vi "Get Communication Specific Objects.vi"(8 "error in":errorcluster, 11 "Electronic Datasheet":refnum<class "Electronic Datasheet.lvclass">) -> (0 "error out":errorcluster, 2 "Entries":refnum<class "OD Entry.lvclass">[](array[class]), 3 "Electronic Datasheet":refnum<class "Electronic Datasheet.lvclass">)   [LabVIEW 2024, in "Electronic Datasheet.lvlib" / "Electronic Datasheet.lvclass"]
uses:
  Electronic Datasheet.lvclass
  Core/OD Entry/OD Entry.lvclass
  Core/Sorted Object Dictionary/Sorted Object Dictionary.lvclass
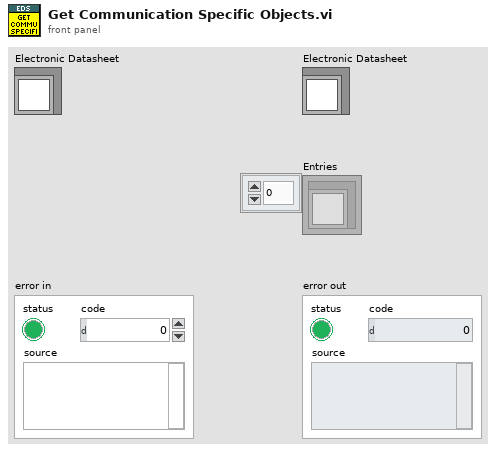
[diagram p1: front panel]
types:
  T1 = typedef "Electronic Datasheet.lvlib/Electronic Datasheet.lvclass/ObjectAttributes.ctl" = cluster{"EDS File Path":path, "Object Dict":refnum<class "Dictionary.lvclass">, "Sorted Object Dict":refnum<class "Sorted Object Dictionary.lvclass">, "Device Info":refnum<class "Device Info.lvclass">, "File Info":refnum<class "File Info.lvclass">}
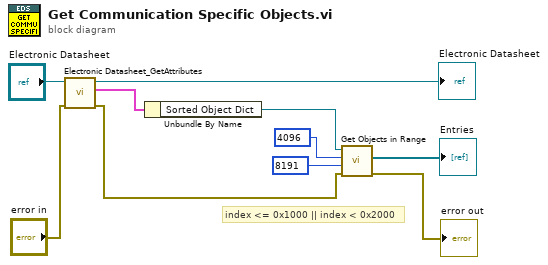
[diagram p0: block diagram]
diagram:
  # "index <= 0x1000 || index < 0x2000"
  n1 = call "Electronic Datasheet_GetAttributes.vi"("Error In"="error in", "reference in"="Electronic Datasheet") -> ("Error Out"=w6:errorcluster, "Data"=w1:T1, "reference out"=→"Electronic Datasheet":refnum<class "Electronic Datasheet.lvclass">)  [unwired: 6 in, 1 out]
  n2 = Unbundle By Name(w1) -> ("Sorted Object Dict"=w2:refnum<class "Sorted Object Dictionary.lvclass">)
  n3 = call "Get Objects in Range.vi"("error in"=w6, "Upper Bound"=u16 8191 ("Lower Bound"), "Lower Bound"=u16 4096, "Sorted Object Dictionary in"=w2) -> ("error out"=→"error out":errorcluster, "Entries"=→"Entries":refnum<class "OD Entry.lvclass">[])  [unwired: 5 in, 1 out]
